vi "I32 Max.vi"() -> (0 "I32 max":i32=2147483647)   [LabVIEW 2021, in "Math.lvlib"]
doc: "2,147,483,647 = 2^31 - 1"
uses:
  Math.lvlib
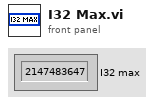
[diagram p1: front panel]
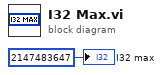
[diagram p0: block diagram]
diagram:
  "I32 max" <- 2147483647 ("Plot Index (Default: Inf, add to end)")
